vi "Get Op Cfg.vi"(8 "error in (no error)":errorcluster, 10 "dummy":bool) -> (0 "error out":errorcluster, 1 "timed out?":bool, 2 "Tool OpCfg":T1={"Use Tool Cfg"=FALSE, "Use Tool Cal"=FALSE, "Fake Data?"=FALSE, "Mode"=-2, "Array Subset Length"=30, "nArrays to Read"=2, "Full Array Read Length"=500, "nSubarrays/Sensor"=0})   [LabVIEW 2015, in "Tool Module.lvlib"]
doc: "Returns the current state of the Tool Module Op Config cluster.\n_____\nCreated using Delacor QMH Event Scripter 2.1.0.3."
uses:
  Tool Module.lvlib
  Tool Config/_Tool Operation Config Cluster--typedef.ctl
  Get Op Cfg Argument--cluster.ctl
  Get Op Cfg (Reply Payload)--cluster.ctl
  Tool Config/Tool Cfg.lvlib
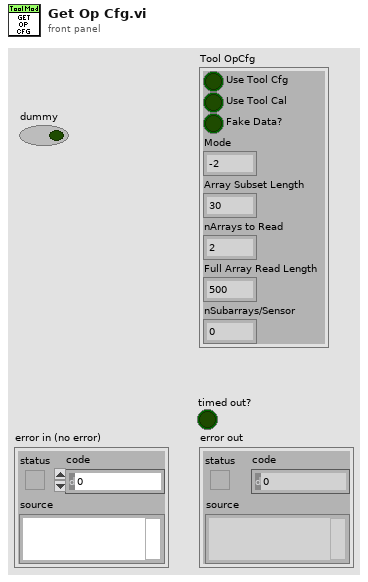
[diagram p1: front panel]
types:
  T1 = typedef "Tool Cfg.lvlib/_Tool Operation Config Cluster--typedef.ctl" = cluster{"Use Tool Cfg":bool, "Use Tool Cal":bool, "Fake Data?":bool, "Mode":i16, "Array Subset Length":i16, "nArrays to Read":i16, "Full Array Read Length":i16, "nSubarrays/Sensor":i16}
  T2 = typedef "Tool Module.lvlib/Get Op Cfg Argument--cluster.ctl" = cluster{"dummy":bool, "Wait Notifier":refnum<notifier>}
  T3 = typedef "Tool Module.lvlib/Request Events--cluster.ctl" = cluster{"Stop Module":refnum<user-event>, "Show Panel":refnum<user-event>, "Hide Panel":refnum<user-event>, "Get Module Execution Status":refnum<user-event>, "Show Diagram":refnum<user-event>, "Set OpCfg":refnum<user-event>, "Get Op Cfg":refnum<user-event>, "Test Trig 2":refnum<user-event>, "GOTO":refnum<user-event>, "Start Inspect":refnum<user-event>, "CONNECT":refnum<user-event>, "Get All Inspect Data":refnum<user-event>, "Get Inspection Limits":refnum<user-event>, "Set Inspection Limits":refnum<user-event>, "Update Status":refnum<user-event>, "Get Data Format Params":refnum<user-event>, "Start Data Monitor":refnum<user-event>, "Get FPGA Setup Params":refnum<user-event>, "Set FPGA Setup Params":refnum<user-event>, "Set Tool Config":refnum<user-event>, "Get Tool Config":refnum<user-event>, "Set Integration Count":refnum<user-event>, "Set Laser Params":refnum<user-event>, "Get Mtrl Ctrl Reg":refnum<user-event>, "Commit Ctrl Reg":refnum<user-event>, "Set Event Logger":refnum<user-event>, "Write to File":refnum<user-event>, "Read from File":refnum<user-event>}
  T4 = typedef "Tool Module.lvlib/Get Op Cfg (Reply Payload)--cluster.ctl" = cluster{"Tool OpCfg":T1}
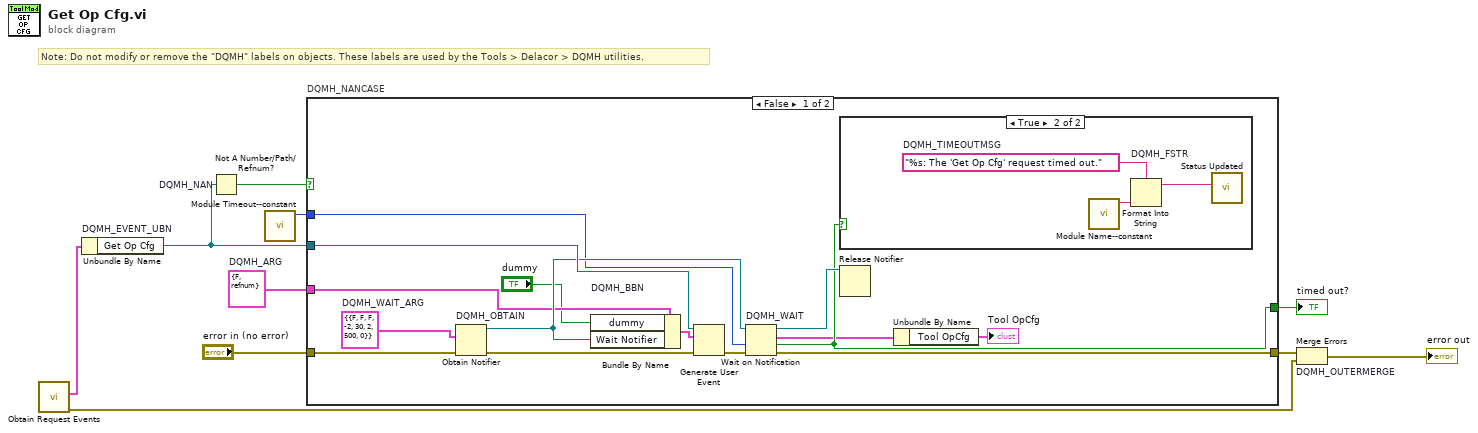
[diagram p0: block diagram]
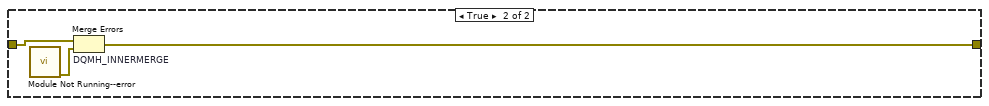
[diagram p3: hidden frame]
diagram:
  w4 = T2 {"dummy"=FALSE, "Wait Notifier"=refnum}  # DQMH_ARG
  # "Note: Do not modify or remove the \"DQMH\" labels on objects. These labels are used by the Tools > Delacor > DQMH utilities."
  n1 = call "Obtain Request Events.vi"() -> ("error out"=w2:errorcluster, "Tool Module Request Events"=w1:T3)  [unwired: 10 in]
  n2 = Unbundle By Name "DQMH_EVENT_UBN"(w1) -> ("Get Op Cfg"=w8:refnum<user-event>)
  n3 = Not A Number/Path/Refnum? "DQMH_NAN"(number/path/refnum=w8) -> (NaN/Path/Refnum?=w7:bool)
  n4 = call "Module Timeout--constant.vi"() -> ("Module Timeout"=w3:i32)  [unwired: 11 in]
  n5 = case "DQMH_NANCASE" shown="False" w7 {
    tunnel: "error in (no error)" -> [w25 w31]
    tunnel: w8 -> [w23 _]
    tunnel: [w20 w30] -> w5
    tunnel: [w17 _] -> w6
    tunnel: w4 -> [w16 _]
    tunnel: w3 -> [w14 _]
    frame False {
      w11 = T4 {"Tool OpCfg"={"Use Tool Cfg"=FALSE, "Use Tool Cal"=FALSE, "Fake Data?"=FALSE, "Mode"=-2, "Array Subset Length"=30, "nArrays to Read"=2, "Full Array Read Length"=500, "nSubarrays/Sensor"=0}}  # DQMH_WAIT_ARG
      n6 = Obtain Notifier "DQMH_OBTAIN"(notification data type=w11, error in (no error)=w25) -> (notifier out=w19:refnum<notifier>, error out=w21:errorcluster)  [unwired: 2 in, 1 out]
      n7 = Bundle By Name "DQMH_BBN"(cluster=w16, "dummy"="dummy", "Wait Notifier"=w19) -> (w22:T2)
      n8 = Generate User Event(user event=w23, event data cluster=w22, error in=w21) -> (error out=w24:errorcluster)  [unwired: 1 in, 1 out]
      n9 = Wait on Notification "DQMH_WAIT"(notifier=w19, timeout in ms (-1)=w14, error in (no error)=w24) -> (notifier out=w18:refnum<notifier>, notification=w13:T4, timed out?=w17:bool, error out=w20:errorcluster)  [unwired: 1 in]
      n10 = case shown="True" w17 {
        frame False {
        }
        frame True {
          w28 = "%s: The 'Get Op Cfg' request timed out."  # DQMH_TIMEOUTMSG
          n11 = call "Module Name--constant.vi"() -> ("Module Name"=w27:string)  [unwired: 11 in]
          n12 = Format Into String "DQMH_FSTR"(format string=w28, w27) -> (resulting string=w26:string)  [unwired: 2 in, 1 out]
          n13 = call "Status Updated.vi"("Status"=w26) -> ()  [unwired: 10 in, 1 out]
        }
      }
      n14 = Release Notifier(notifier=w18) -> ()  [unwired: 2 in, 3 out]
      n15 = Unbundle By Name(w13) -> ("Tool OpCfg"=→"Tool OpCfg":T1)
    }
    frame True {
      n16 = call "Module Not Running--error.vi"() -> ("error out"=w29:errorcluster)  [unwired: 11 in]
      n17 = Merge Errors "DQMH_INNERMERGE"(w31, w29) -> (w30:errorcluster)
    }
  }
  "timed out?" <- w6
  n18 = Merge Errors "DQMH_OUTERMERGE"(w5, w2) -> (→"error out":errorcluster)
